vi "Flatten.vi"(8 "error in (no error)":errorcluster, 11 "Magnetic Field in":refnum<class "Magnetic Field.lvclass">) -> (0 "error out":errorcluster, 3 "Magnetic Field out":refnum<class "Magnetic Field.lvclass">)   [LabVIEW 2012, in "Magnetic Field.lvclass"]
uses:
  Magnetic Field.lvclass
  Scanner/Scanner.lvclass
  Magnetic Field.lvclass/Magnetic Field.ctl
  Global/File Locations.vi
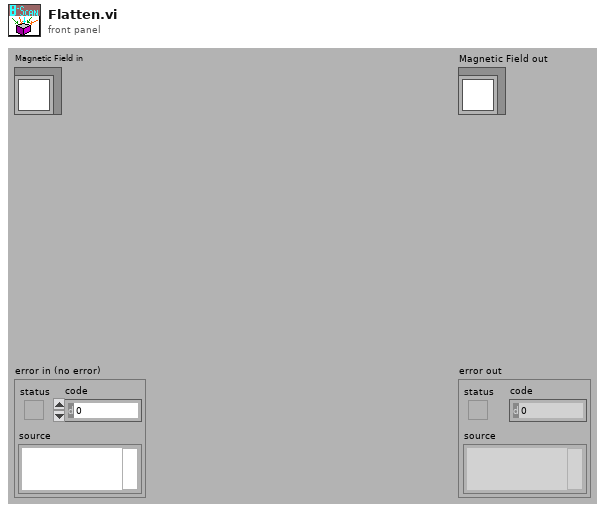
[diagram p1: front panel]
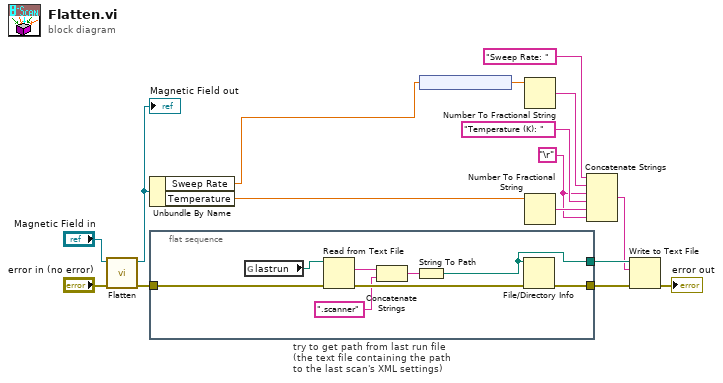
[diagram p0: block diagram]
diagram:
  w2 = "\r"
  n1 = call-parent "Flatten.vi"("error in (no error)"="error in (no error)", "Scanner in"="Magnetic Field in") -> ("error out"=w13:errorcluster, "Scanner out"=w14:refnum<class "Magnetic Field.lvclass">)  [unwired: 8 in]
  "Magnetic Field out" <- w14
  n2 = Unbundle By Name(w14) -> ("Sweep Rate"=w8:dbl[unit], "Temperature"=w9:dbl)
  n3 = flat-sequence "try to get path from last run file\n(the text file containing the path\nto the last scan's XML settings)" {
    tunnel: [w24] -> w10
    tunnel: [w21] -> w11
    tunnel: w13 -> [w20]
    frame #0 {
      n4 = global read "File Locations.vi" "lastrun"() -> (w23:path)
      n5 = Read from Text File(file (use dialog)=w23, error in=w20) -> (text=w19:string, error out=w22:errorcluster)  [unwired: 4 out]
      n6 = Concatenate Strings(w19, ".scanner") -> (w17:string)
      n7 = String To Path(string=w17) -> (path=w24:path)
      n8 = File/Directory Info(path=w24, error in=w22) -> (error out=w21:errorcluster)  [unwired: 6 out]
    }
  }
  n9 = node(w8) -> (w7:dbl)
  n10 = Number To Fractional String(number=w7) -> (F-format string=w5:string)  [unwired: 3 in]
  n11 = Number To Fractional String(number=w9) -> (F-format string=w3:string)  [unwired: 3 in]
  n12 = Concatenate Strings("Sweep Rate: ", w5, w2, "Temperature (K): ", w3, w2) -> (w1:string)
  n13 = Write to Text File(file (use dialog)=w10, text=w1, error in=w11) -> (error out=→"error out":errorcluster)  [unwired: 1 in, 2 out]
